vi "Configure Channel (Slop).vi"(7 "Event Type (1: Start)":i32(ring)=1 items=["Start"=1, "Stop"=2], 8 "error in (no error)":errorcluster, 9 "Active Edge (1: Negative)":i32(ring)=1 items=["Positive", "Negative"], 10 "Channel (1: Channel 1)":i32(ring)=1 items=["Channel 1"=1, "Channel 2"=2], 11 "VISA resource name":refnum<visa-resource-name>) -> (0 "error out":errorcluster, 3 "VISA resource name out":refnum<visa-resource-name>)   [LabVIEW 2024, in "Agilent 532XX Series.lvlib"]
doc: "Selects the active edge of the input signal that will be used for measurements."
uses:
  Agilent 532XX Series.lvlib
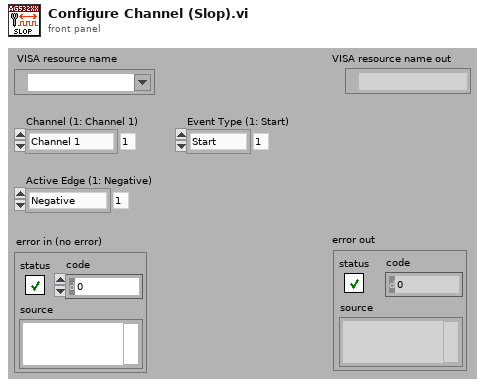
[diagram p1: front panel]
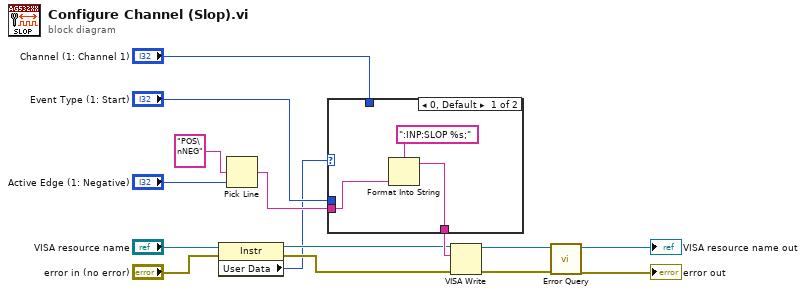
[diagram p0: block diagram]
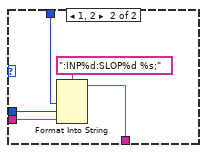
[diagram p2: hidden frame]
diagram:
  n1 = property class="Instr"(reference="VISA resource name", error in="error in (no error)") -> (reference out=w3:refnum<visa-resource-name>, error out=w2:errorcluster, "User Data"=w1:u32)
  n2 = Pick Line(multi-line string="POS\nNEG", line index="Active Edge (1: Negative)") -> (output string=w11:string)  [unwired: 1 out]
  n3 = case shown="0, Default" w1 {
    tunnel: "Channel (1: Channel 1)" -> [_ w22]
    tunnel: "Event Type (1: Start)" -> [_ w21]
    tunnel: w11 -> [w17 w20]
    tunnel: [w16 w19] -> w10
    frame 0, Default {
      n4 = Format Into String(format string=":INP:SLOP %s;", w17) -> (resulting string=w16:string)  [unwired: 2 in, 1 out]
    }
    frame 1, 2 {
      n5 = Format Into String(format string=":INP%d:SLOP%d %s;", w22, w21, w20) -> (resulting string=w19:string)  [unwired: 2 in, 1 out]
    }
  }
  n6 = VISA Write(VISA resource name=w3, write buffer=w10, error in (no error)=w2) -> (VISA resource name out=w9:refnum<visa-resource-name>, error out=w8:errorcluster)  [unwired: 1 out]
  n7 = call "Error Query.vi"("error in (no error)"=w8, "VISA resource name"=w9) -> ("error out"=→"error out":errorcluster, "VISA resource name out"=→"VISA resource name out":refnum<visa-resource-name>)  [unwired: 8 out]
